vi "Lockin_Example_IV_Curves.vi"() -> ()   [LabVIEW 2016]
uses:
  Typedefs/AO-cluster.ctl
  Typedefs/AO_Amp-array.ctl
  Typedefs/AO_DC-array.ctl
  Typedefs/AO_f-array.ctl
  Typedefs/AO_phi-array.ctl
  Typedefs/Function-array.ctl
  Typedefs/Function-enum.ctl
  <userlib>/LevyLab/LV to ITX/LVtoITX.lvclass
panel:
  out "2 terminal":cluster{"Y":dbl[], "Y":dbl[]}(graph)
  out "4 terminal":cluster{"Y":dbl[], "Y":dbl[]}(graph)
  in  "step":dbl=0.025
  in  "end":dbl=0.1
  in  "start":dbl
  in  "Channels: AO":T1={"AO amp (V)"=[0.1, 0.2, 0.0, 0.0, 0.0, 0.0, 0.0, 0.0], "AO DC (V)"=[0.0, 0.0, 0.0, 0.0, 0.0, 0.0, 0.0, 0.0], "AO f (Hz)"=[1.0, 1.0, 1.0, 1.0, 1.0, 1.0, 1.0, 1.0], "AO phi (deg)"=[0.0, 0.0, 0.0, 0.0, 0.0, 0.0, 0.0, 0.0], "function"=[enum."Triangle Wave", enum."Triangle Wave", enum."Sine Wave", enum."Sine Wave", enum."Sine Wave", enum."Sine Wave", enum."Sine Wave", enum."Sine Wave"]} {"AO f (Hz)" min=0.001 max=10000.0; "AO DC (V)" format="%#_6p"; "AO amp (V)" format="%#_6p"}
  # "Lockin Example: IV Curves\nMake Sure Lockin Program is running!"
  # "0"
  # "1"
  # "2"
  # "3"
  # "4"
  # "5"
  # "6"
  # "7"
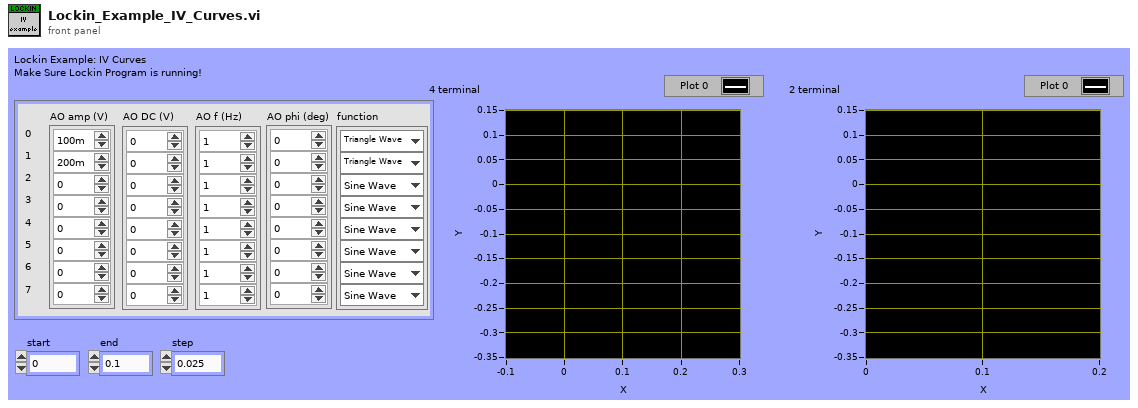
[diagram p1: front panel]
types:
  T1 = typedef "AO-cluster.ctl" = cluster{"AO amp (V)":T2, "AO DC (V)":T3, "AO f (Hz)":T4, "AO phi (deg)":T5, "function":T6}
  T2 = typedef "AO_Amp-array.ctl" = dbl[]
  T3 = typedef "AO_DC-array.ctl" = dbl[]
  T4 = typedef "AO_f-array.ctl" = dbl[]
  T5 = typedef "AO_phi-array.ctl" = dbl[]
  T6 = typedef "Function-array.ctl" = T7[]
  T7 = typedef "Function-enum.ctl" = enum16{"Sine Wave", "Triangle Wave", "Square Wave", "Sawtooth Wave"}
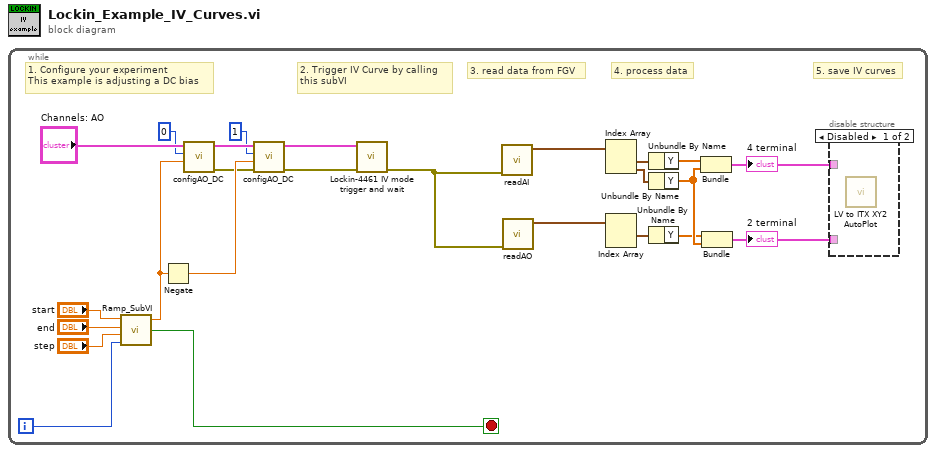
[diagram p0: block diagram]
diagram:
  n1 = while {
    i -> [w22]
    stop <- w25 stop-if-true
    # "5. save IV curves"
    # "4. process data"
    # "3. read data from FGV"
    # "1. Configure your experiment\nThis example is adjusting a DC bias"
    # "2. Trigger IV Curve by calling\nthis subVI"
    n2 = call <userlib>:"Ramp_SubVI.vi"("index"=w22, "step"="step", "end"="end", "start"="start") -> ("Stop?"=w25:bool, "Numeric"=w6:dbl)  [unwired: 1 in]
    n3 = Negate(x=w6) -> (-x=w5:dbl)
    n4 = call "configAO_DC.vi"("new DC (V)"=w6, "AO Channel"=0, "Channels: AO"="Channels: AO") -> ("error out"=w2:errorcluster, "Channels: AO"=w8:T1)  [unwired: 7 in]
    n5 = call "configAO_DC.vi"("error in (no error)"=w2, "new DC (V)"=w5, "AO Channel"=1, "Channels: AO"=w8) -> ("error out"=w1:errorcluster, "Channels: AO"=w7:T1)  [unwired: 6 in]
    n6 = call "Lockin-4461 IV mode trigger and wait.vi"("error in (no error)"=w1, "Channels: AO"=w7) -> ("error out"=w11:errorcluster)  [unwired: 9 in]
    n7 = call "readAI.vi"("error in (no error)"=w11) -> ("input signal"=w12:waveform(dbl)[])  [unwired: 9 in, 1 out]
    n8 = call "readAO.vi"("error in (no error)"=w11) -> ("output signal"=w10:waveform(dbl)[])  [unwired: 9 in, 1 out]
    n9 = Index Array(array=w12) -> (element #1=w20:waveform(dbl), element #2=w18:waveform(dbl))  [unwired: 2 in]
    n10 = Index Array(array=w10) -> (element #1=w17:waveform(dbl))  [unwired: 2 in, 1 out]
    n11 = Unbundle By Name(w20) -> ("Y"=w19:dbl[])
    n12 = Unbundle By Name(w18) -> ("Y"=w16:dbl[])
    n13 = Unbundle By Name(w17) -> ("Y"=w15:dbl[])
    n14 = Bundle("Y"=w19, "Y"=w16) -> (w14:cluster{"Y":dbl[], "Y":dbl[]})  [unwired: 1 in]
    "4 terminal" <- w14
    n15 = Bundle("Y"=w15, "Y"=w16) -> (w13:cluster{"Y":dbl[], "Y":dbl[]})  [unwired: 1 in]
    "2 terminal" <- w13
    n16 = disable-structure shown="Disabled" {
      disable-tunnel: w14 -> [_ _]
      disable-tunnel: w13 -> [_ _]
      frame Disabled {
        n17 = call <userlib>:"LV to ITX XY2 AutoPlot.vi"() -> ()  [unwired: 15 in, 1 out]
      }
      frame Enabled {
      }
    }
  }
